vi "UDP Multicast Receiver.vi"() -> ()   [LabVIEW 2010]
doc: "Demonstrates how to work with the UDP Multicast Sender.vi. Run this VI first.\n\nUDP multicast will allow LabVIEW to send data to a multicast group or to receive data sent to a multicast group. In LabVIEW, UDP multicast is used in very much the same way as UDP. The main difference is there are two new parameters, TTL and Multicast Address, on the UDP Multicast Open. \n\nWhen sending to a multicast group the default time-to-live (TTL) is 1, which only allows the packet to go to the local subnet. When a router receives a multicast packet, it decrements the packets TTL, and if the TTL is greater than 0, forwards the packet to other routers.\nA multicast group is defined by having a multicast IP address in the range 224.0.0.0 to 239.255.255.255."
uses:
  <vilib>/Utility/tcp.llb/UDP Multicast Open.vi
  <vilib>/addons/internet/NI_InternetTK_Common_VIs.lvlib
panel:
  in  "stop":bool
  in  "Multicast Address":string="234.5.6.7"
  in  "Port":i32=58432
  out "Data Received":string
  # "Instructions:\n1. Open the UDP Multicast Sender.vi located in the same library.\n2. Make sure that Port in this VI and Send to Port in the UDP Multicast Sender.vi are the same and that they have the same Multicast Address.\n3. Run this VI first\n4. Run the UDP Multicast Sender VI second\nNote: This VI is built to work with the UDP Multicast Sender.vi."
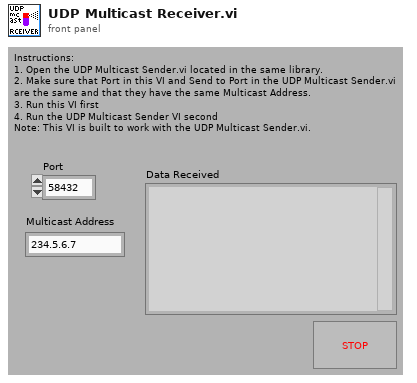
[diagram p1: front panel]
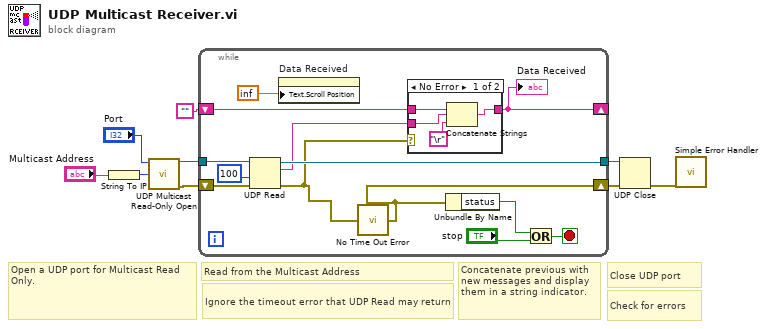
[diagram p0: block diagram]
diagram:
  # "Open a UDP port for Multicast Read Only."
  # "Read from the Multicast Address"
  # "Close UDP port"
  # "Check for errors"
  # "Concatenate previous with new messages and display them in a string indicator."
  # "Ignore the timeout error that UDP Read may return"
  n1 = String To IP(1:"Multicast Address") -> (0:w6:u32)
  n2 = call-poly <vilib>:"UDP Multicast Read-Only Open.vi"("multicast addr"=w6, "port"="Port") -> ("error out"=w7:errorcluster, "connection ID"=w9:refnum<k16>)  [unwired: 2 in, 6 out]
  n3 = while {
    tunnel: w9 -> [w21]
    tunnel: [w22] -> w8
    shift-right: [w19] -> _
    shift-left: "" -> [w20]
    shift-right: [w10] -> w1
    shift-left: w7 -> [w14]
    stop <- w16 stop-if-true
    n4 = UDP Read(connection ID=w21, timeout ms (25000)=100, 8:w14) -> (data out=w13:string, error out=w11:errorcluster, 3:w22:refnum<k16>)  [unwired: 3 out]
    n5 = property on="Data Received" class="Str"("Text.Scroll Position"=inf) -> ()  [unwired: 2 in, 2 out]
    n6 = call <vilib>:"No Time Out Error.vi"("error in (no error)"=w11) -> ("error out"=w10:errorcluster)  [unwired: 14 in]
    n7 = case shown="No Error" w11 {
      tunnel: w20 -> [w26 w27]
      tunnel: w13 -> [w23 _]
      tunnel: [w24 w27] -> w19
      frame No Error {
        n8 = Concatenate Strings(w26, w23, "\r") -> (w24:string)
      }
      frame Error {
      }
    }
    "Data Received" <- w19
    n9 = Unbundle By Name(w10) -> ("status"=w18:bool)
    n10 = Or(x=w18, y="stop") -> (x .or. y?=w16:bool)
  }
  n11 = UDP Close(connection ID=w8, 8:w1) -> (error out=w4:errorcluster)  [unwired: 1 out]
  n12 = call <vilib>:"Simple Error Handler.vi"("error in (no error)"=w4) -> ()  [unwired: 1 in, 8 out]
